vi "RefNums_Sensors.vi"() -> ()   [LabVIEW 2018]
panel:
  out "Ground_Prox_Sensor":string
  out "Upper_Pressure_Transducer":string
  out "Tank_Pressure_Transducer":string
  out "Accelerometer":string
  out "Front_Left_Prox_Sensor":string
  out "Front_Right_Prox_Sensor":string
  out "Rear_Prox_Sensor":string
  out "Left_Prox_Sensor":string
  out "Right_Prox_Sensor":string
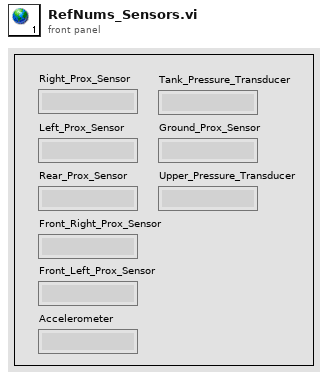
[diagram p1: front panel]
diagram:
